vi "Throttle.vi"(9 "Atmospheric Pressure (bar)":sgl, 10 "Manifold Pressure (bar)":sgl, 11 "Throttle Angle (deg)":sgl) -> (2 "Throttle Flow (g/s)":sgl)   [LabVIEW 2016, in "NI-PCG Vehicle Model.lvlib"]
uses:
  NI-PCG Vehicle Model.lvlib
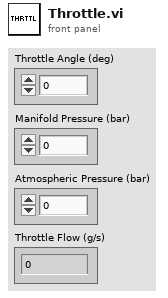
[diagram p1: front panel]
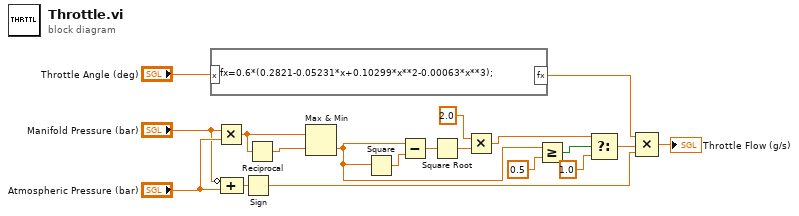
[diagram p0: block diagram]
diagram:
  n1 = formula code="fx=0.6*(0.2821-0.05231*x+0.10299*x**2-0.00063*x**3);"("x"="Throttle Angle (deg)") -> ("fx"=w1:dbl)
  n2 = Multiply(x="Manifold Pressure (bar)", y="Atmospheric Pressure (bar)") -> (x*y=w19:sgl)
  n3 = Compound Arithmetic op=ADD(invert "Manifold Pressure (bar)", "Atmospheric Pressure (bar)") -> (w15:sgl)
  n4 = Sign(1:w15) -> (0:w10:sgl)
  n5 = Reciprocal(x=w19) -> (1/x=w18:sgl)
  n6 = Max & Min(x=w19, y=w18) -> (min(x,y)=w3:sgl)  [unwired: 1 out]
  n7 = Square(x=w3) -> (x^2=w14:sgl)
  n8 = Subtract(x=w3, y=w14) -> (x-y=w13:sgl)
  n9 = Square Root(x=w13) -> (sqrt(x)=w12:sgl)
  n10 = Multiply(x=sgl 2.0, y=w12) -> (x*y=w8:sgl)
  n11 = Greater Or Equal?(x=w3, y=sgl 0.5) -> (x >= y?=w6:bool)
  n12 = Select(t=w8, s=w6, f=sgl 1.0) -> (s? t:f=w7:sgl)
  n13 = Compound Arithmetic op=MULTIPLY(w1, w7, w10) -> (→"Throttle Flow (g/s)":dbl)
